vi "toggleinput.vi"(11 "Boolean":bool) -> (3 "Boolean 2":bool)   [LabVIEW 2016]
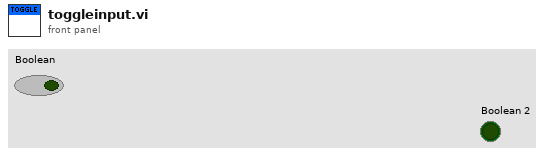
[diagram p1: front panel]
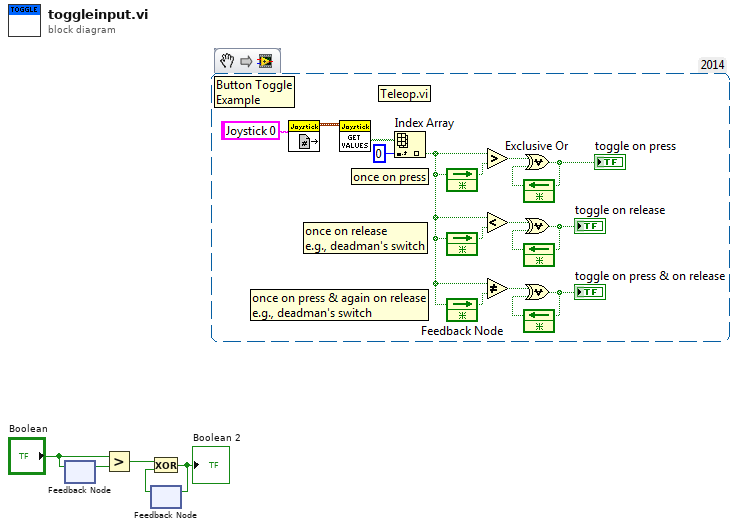
[diagram p0: block diagram]
diagram:
  n1 = feedback #1() -> (w2:bool)  [unwired: 1 in]
  n2 = feedback-in #1("Boolean") -> ()
  n3 = Greater?(x="Boolean", y=w2) -> (0:w3:bool)
  n4 = feedback #2() -> (w5:bool)  [unwired: 1 in]
  n5 = Exclusive Or(1:w5, 2:w3) -> (0:w4:bool)
  "Boolean 2" <- w4
  n6 = feedback-in #2(w4) -> ()
